vi "test High Priority SubRoutines.vi"(8 "error in (no error)":errorcluster, 11 "BC Async SubRoutines in":refnum<class "BC Async SubRoutines.lvclass">) -> (0 "error out":errorcluster, 3 "BC Async SubRoutines out":refnum<class "BC Async SubRoutines.lvclass">)   [LabVIEW 2016, in "BC Async SubRoutines.lvclass"]
uses:
  BC Async SubRoutines.lvclass
  BCI-1553 API.lvlib
  Frames & Messages/TypeDefs/BC Op Codes - Verbose.ctl
  Frames & Messages/TypeDefs/BC Condition Codes.ctl
  PPLs/FPGA Interface.lvlibp/FPGA Interface/FPGA Interface.lvclass
panel:
  out "Arb Addr":u16 format="%04x"
  out "Data":u16[](array[numeric]) format="%04x"
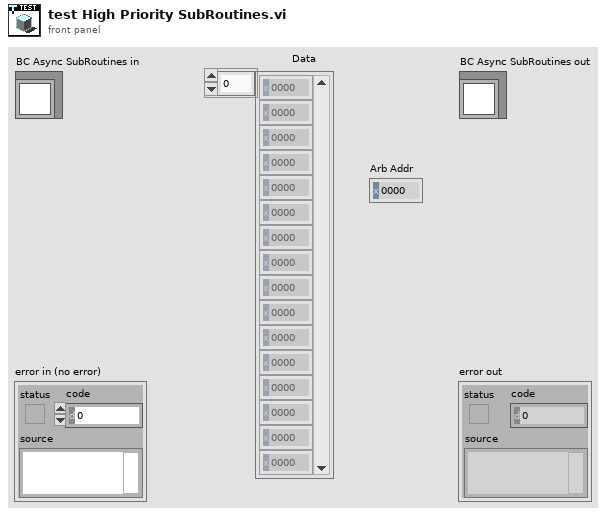
[diagram p1: front panel]
types:
  T1 = typedef "BCI-1553 API.lvlib/BC Condition Codes.ctl" = enum16{"GP0 == 1 || LT", "GP1 == 1 || NE", "GP2 == 1", "GP3 == 1", "GP4 == 1", "GP5 == 1", "GP6 == 1", "GP7 == 1", "NORESP", "FMTERR", "GOODBLOCK", "MSKSTATSET", "BADMSG", "1RETRY", "2RETRY", "ALWAYS"}
  T2 = typedef "BCI-1553 API.lvlib/BC Op Codes - Verbose.ctl" = enum16{"EXECUTE MSG", "EXECUTE MSG GO", "JUMP", "CALL SUBROUTINE", "RETURN", "INTERRUPT REQUEST", "HALT", "DELAY", "WAIT FRAME TIMER = 0", "COMPARE FRAME TIMER", "COMPARE MSG TIMER", "LOAD TIME TAG CTR", "LOAD TIME TAG CTR HI", "LOAD FRAME TIMER", "START FRAME TIMER", "PUSH TIME TAG COUNT", "PUSH TIME TAG COUNT HI", "PUSH TIME TAG COUNT BOTH", "PUSH BLOCK STATUS WORD", "PUSH CURRENT VALUE", "PUSH INDIRECT", "WAIT EXT TRIGGER", "EXECUTE AND FLIP", "EXECUTE, FLIP, GO", "WRITE VALUE TO WMI", "WRITE VALUE TO MEM", "DECREMENT RAM, SKIP", "FLAG"}
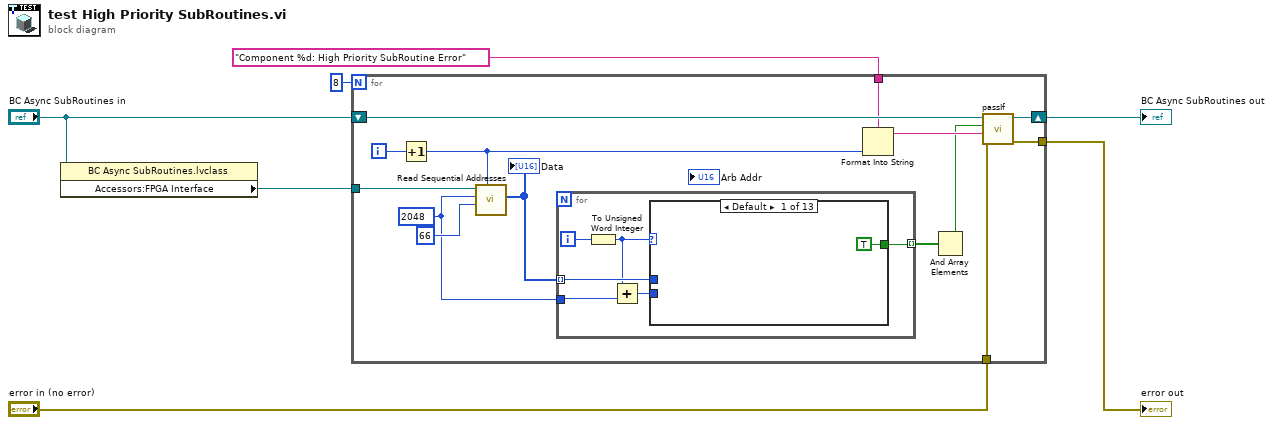
[diagram p0: block diagram]
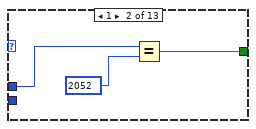
[diagram p2: hidden frame]
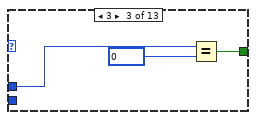
[diagram p3: hidden frame]
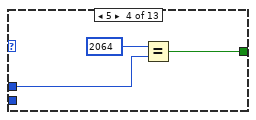
[diagram p4: hidden frame]
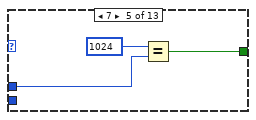
[diagram p5: hidden frame]
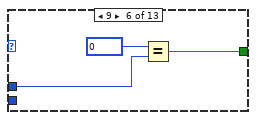
[diagram p6: hidden frame]
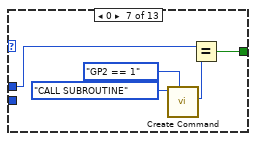
[diagram p7: hidden frame]
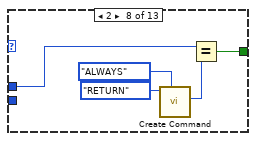
[diagram p8: hidden frame]
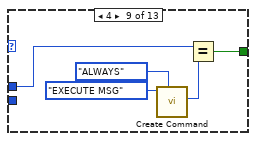
[diagram p9: hidden frame]
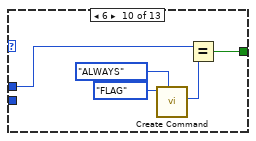
[diagram p10: hidden frame]
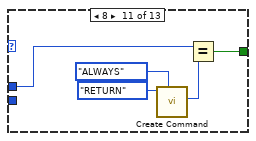
[diagram p11: hidden frame]
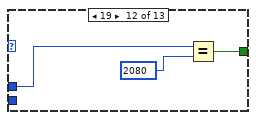
[diagram p12: hidden frame]
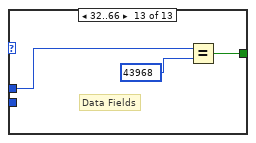
[diagram p13: hidden frame]
diagram:
  n1 = property class="BC Async SubRoutines.lvclass"(reference="BC Async SubRoutines in") -> ("Accessors:FPGA Interface"=w7:refnum<class "FPGA Interface.lvclass">)  [unwired: 1 in, 2 out]
  n2 = for {
    N: 8 -> [_]
    tunnel: w7 -> [w21]
    shift-right: [w18] -> w2
    shift-left: "BC Async SubRoutines in" -> [w19]
    tunnel: "error in (no error)" -> [w17]
    tunnel: [w16] -> w3
    tunnel: "Component %d: High Priority SubRoutine Error" ("custom report message (\"\")") -> [w15]
    i -> [w20]
    w8 = u16 2048
    n3 = Increment(x=w20) -> (x+1=w12:i32)
    n4 = call-dynamic "Read Sequential Addresses.vi"("Target IC (1-8)"=w12, "Addresses to Read"=u16 66, "Starting Address"=w8, "FPGA Interface in"=w21) -> ("Data"=w11:u16[])  [unwired: 6 in, 1 out]
    "Data" <- w11
    n5 = for {
      tunnel: w11 -> [w26] mode=indexing
      tunnel: [w27] -> w10 mode=indexing
      tunnel: w8 -> [w25]
      i -> [w24]
      n6 = To Unsigned Word Integer(number=w24) -> (unsigned 16bit integer=w22:u16)
      n7 = Add(x=w22, y=w25) -> (x+y=w23:u16)
      n8 = case shown="Default" w22 {
        tunnel: [TRUE w29 w34 w37 w40 w43 w45 w50 w55 w60 w65 w71 w74] -> w27
        tunnel: w26 -> [_ w31 w33 w35 w38 w41 w44 w49 w54 w59 w64 w69 w72]
        tunnel: w23 -> [_ _ _ _ _ _ _ _ _ _ _ _ _]
        frame Default {
        }
        frame 1 {
          n9 = Equal?(x=w31, y=u16 2052) -> (x = y?=w29:bool)
        }
        frame 3 {
          n10 = Equal?(x=w33, y=u16 0) -> (x = y?=w34:bool)
        }
        frame 5 {
          n11 = Equal?(x=u16 2064, y=w35) -> (x = y?=w37:bool)
        }
        frame 7 {
          n12 = Equal?(x=u16 1024, y=w38) -> (x = y?=w40:bool)
        }
        frame 9 {
          n13 = Equal?(x=u16 0, y=w41) -> (x = y?=w43:bool)
        }
        frame 0 {
          n14 = call "Create Command.vi"("Condition"=BC_Condition_Codes."GP2 == 1", "Op Code"=BC_Op_Codes_-_Verbose."CALL SUBROUTINE") -> ("Instruction"=w46:u16)  [unwired: 8 in, 1 out]
          n15 = Equal?(x=w44, y=w46) -> (x = y?=w45:bool)
        }
        frame 2 {
          n16 = call "Create Command.vi"("Condition"=BC_Condition_Codes."ALWAYS", "Op Code"=BC_Op_Codes_-_Verbose."RETURN") -> ("Instruction"=w51:u16)  [unwired: 8 in, 1 out]
          n17 = Equal?(x=w49, y=w51) -> (x = y?=w50:bool)
        }
        frame 4 {
          n18 = call "Create Command.vi"("Condition"=BC_Condition_Codes."ALWAYS", "Op Code"=BC_Op_Codes_-_Verbose."EXECUTE MSG") -> ("Instruction"=w56:u16)  [unwired: 8 in, 1 out]
          n19 = Equal?(x=w54, y=w56) -> (x = y?=w55:bool)
        }
        frame 6 {
          n20 = call "Create Command.vi"("Condition"=BC_Condition_Codes."ALWAYS", "Op Code"=BC_Op_Codes_-_Verbose."FLAG") -> ("Instruction"=w61:u16)  [unwired: 8 in, 1 out]
          n21 = Equal?(x=w59, y=w61) -> (x = y?=w60:bool)
        }
        frame 8 {
          n22 = call "Create Command.vi"("Condition"=BC_Condition_Codes."ALWAYS", "Op Code"=BC_Op_Codes_-_Verbose."RETURN") -> ("Instruction"=w66:u16)  [unwired: 8 in, 1 out]
          n23 = Equal?(x=w64, y=w66) -> (x = y?=w65:bool)
        }
        frame 19 {
          n24 = Equal?(x=w69, y=u16 2080) -> (x = y?=w71:bool)
        }
        frame 32..66 {
          # "Data Fields"
          n25 = Equal?(x=w72, y=u16 43968) -> (x = y?=w74:bool)
        }
      }
    }
    n26 = Format Into String(format string=w15, w12) -> (resulting string=w14:string)  [unwired: 2 in, 1 out]
    n27 = And Array Elements(Boolean array=w10) -> (logical AND=w9:bool)
    n28 = call-dynamic "passIf.vi"("error in (no error)"=w17, "message (\"\")"=w14, "pass"=w9, "TestCase in"=w19) -> ("error out"=w16:errorcluster, "TestCase out"=w18:refnum<class "BC Async SubRoutines.lvclass">)  [unwired: 6 in]
  }
  "error out" <- w3
  "BC Async SubRoutines out" <- w2
